vi "_Main.vi"   [LabVIEW 2017, in "SRX SubSystem.lvlib"]
uses:
  SRX SubSystem.lvlib
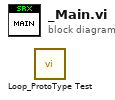
[diagram p0: block diagram]
diagram:
  n1 = call "Loop_ProtoType Test.vi"() -> ()  [unwired: 12 in]
